vi "Lens voltage control (temp).vi"() -> ()   [LabVIEW 2018]
uses:
  <vilib>/Analysis/NI_AALBase.lvlib
  <vilib>/Analysis/baseanly.llb/Mean (DBL).vi
  <vilib>/Utility/file.llb/Write Delimited Spreadsheet (DBL).vi
panel:
  out "Scan Rate (Hz)":dbl=60.0
  out "Error Message":string
  out "Actual ScanRate":dbl format="%.3f"
  out "size(s)":i32[](array[numeric])
  out "Voltage divider 2 (V)":dbl
  out "Voltage divider 1 (V)":dbl
  in  "Active":bool
  out "Initial time":dbl
  in  "Save data path":path=path "C:/Documents and Settings/EDM/Desktop/all_cond_argon_20kV_1x10-4.txt"
  in  "Save data?":bool=TRUE caption="Enable"
  out "Supply 2 Current":waveform(dbl)(graph)
  out "Supply 1 Current":waveform(dbl)(graph)
  out "Supply 2 Voltage":waveform(dbl)(graph)
  out "Waveform Chart":dbl(graph)
  out "Loop iteration time":dbl
  in  "PS2 Set Voltage (kV)":dbl min=0.0 max=30.01 step=0.1 format="%.3f"
  in  "Both power supplies at\nsame voltage? (If true, \nPS1 voltage controls both supplies)":bool
  in  "Ramp time (s)":dbl
  out "relative seconds":dbl format="%_19f"
  out "time string":string
  out "date string":string
  in  "Polarity switch 2 (ON = pos)":bool
  in  "Polarity switch 1 (ON = pos)":bool
  in  "POWER":bool
  in  "Stop":bool
  out "PS2 Voltage (kV)":dbl
  out "PS1 Voltage (kV)":dbl
  in  "PS1 Set Voltage (kV)":dbl min=0.0 max=30.01 step=0.1 format="%.3f"
  out "Ramp Step Size (kV)":dbl=0.025
  in  "Ramp Threshold (kV)":dbl=0.025
  in  "Ramp Voltage?":bool
  out "Supply 1 Voltage":waveform(dbl)(graph)
  out "DeviceScanBacklog":i32
  out "LJMScanBacklog":i32=10
  out "Run Time":string="0  00:02:11" caption="Elapsed Time Text"
  out "Number of\nChannels":i32
  out "ScansPerRead":i32
  in  "Channels to Scan":string[](array[string])=["AIN0", "AIN1", "AIN2", "AIN3", "AIN4", "AIN5", "AIN6", "AIN7", "AIN8", "AIN9", "AIN10", "AIN11", "AIN12", "AIN13"]
  in  "Device type":string(combo)="Ethernet"
  in  "Connection Type":string(combo)="Ethernet"
  out "Connection Error on Start?":bool
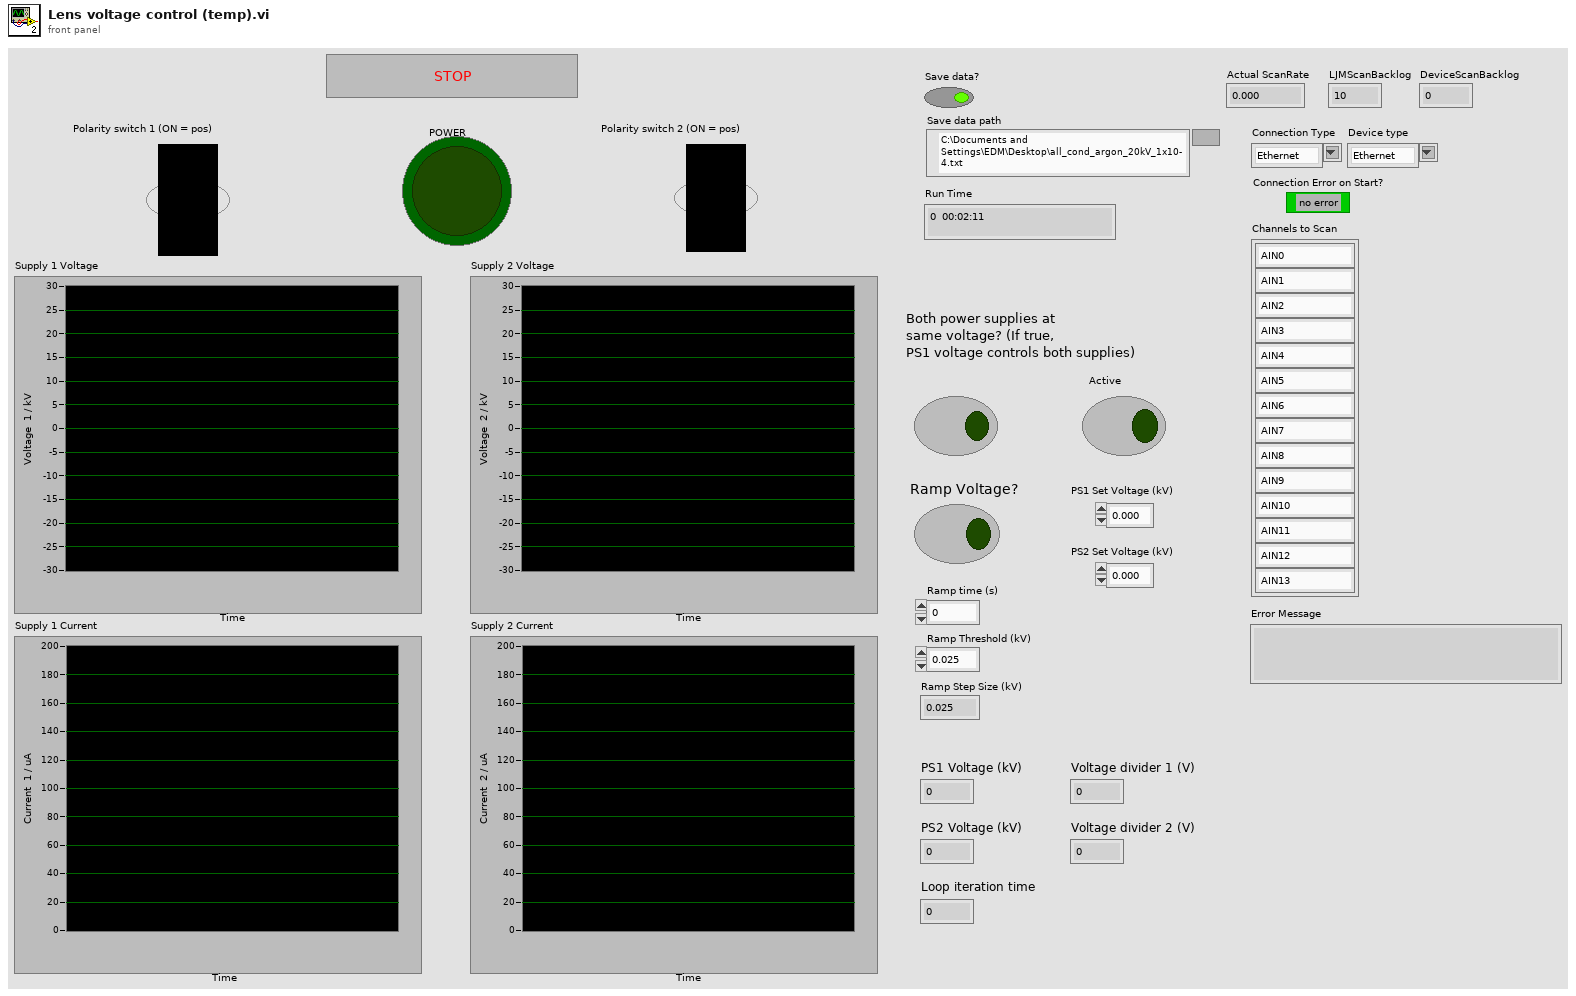
[diagram p1: front panel]
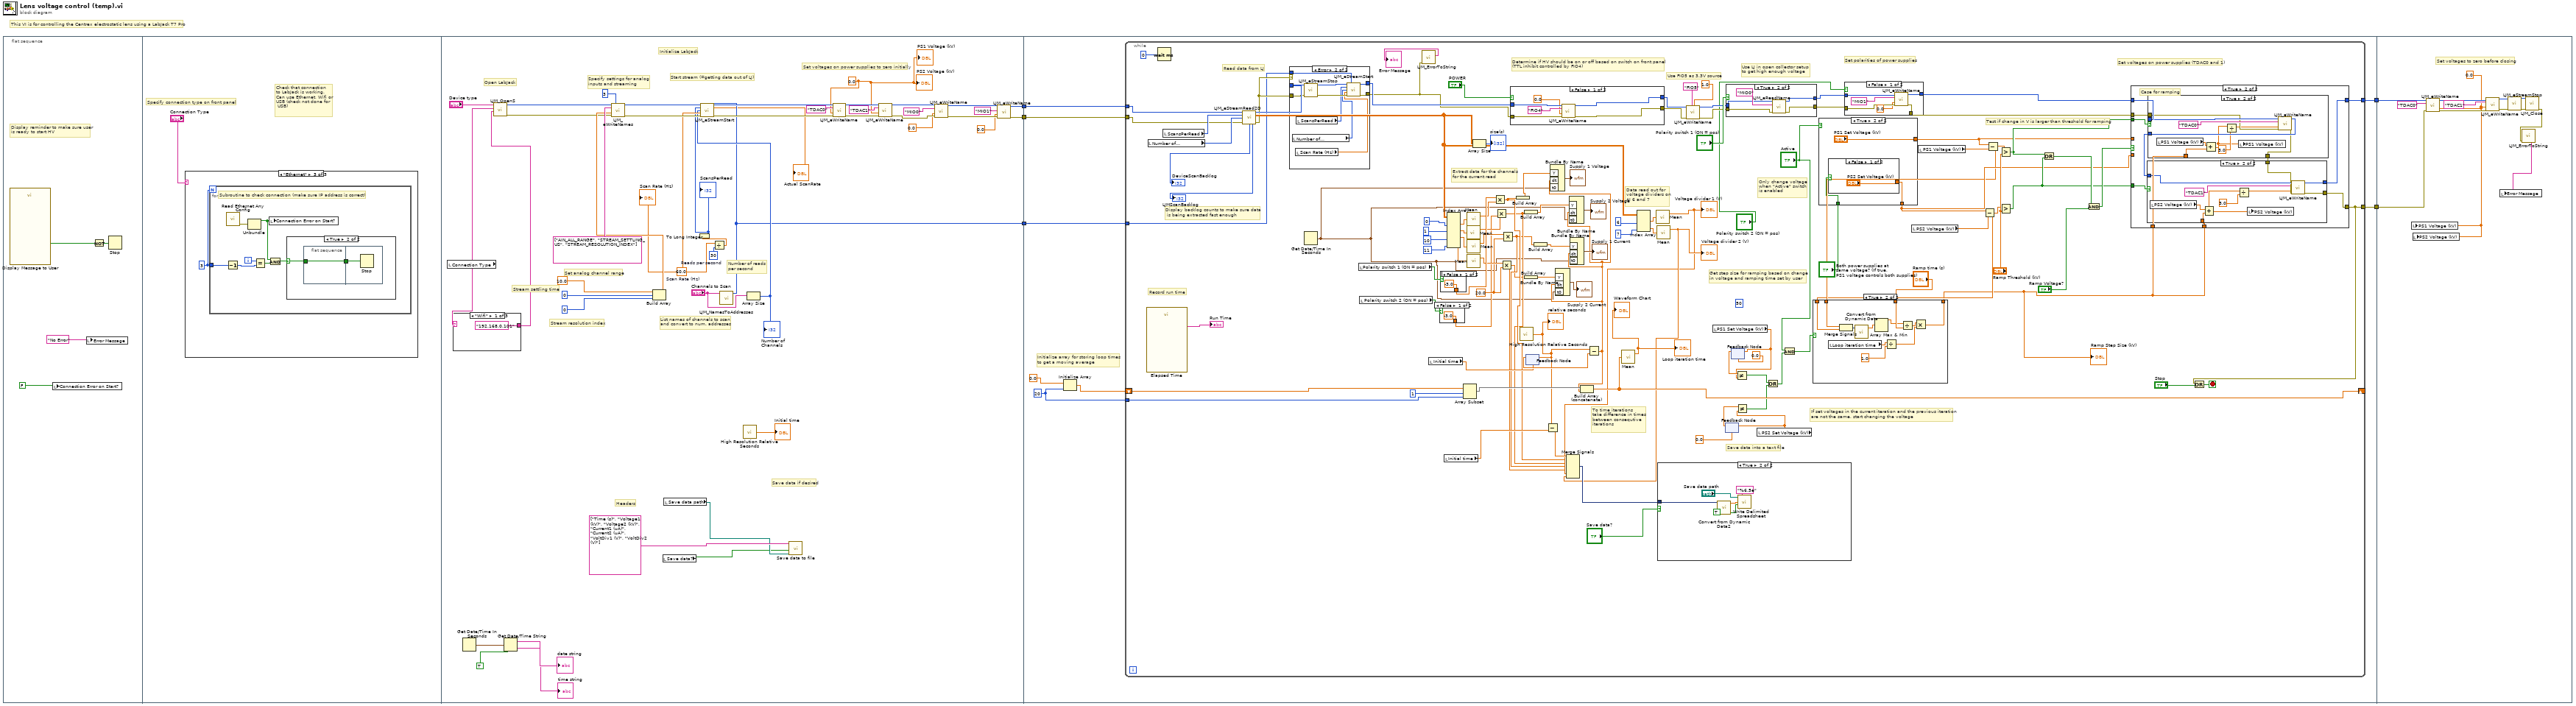
[diagram p0: block diagram]
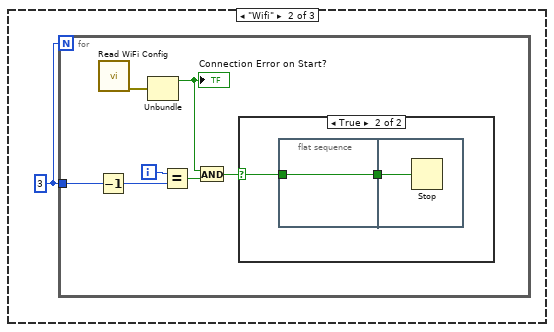
[diagram p3: hidden frame]
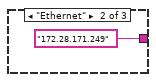
[diagram p6: hidden frame]
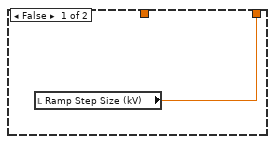
[diagram p9: hidden frame]
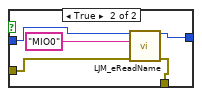
[diagram p10: hidden frame]
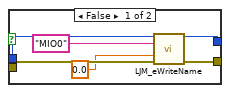
[diagram p11: hidden frame]
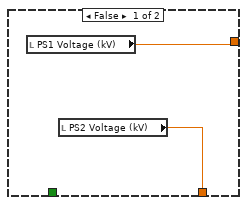
[diagram p12: hidden frame]
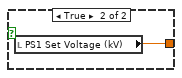
[diagram p13: hidden frame]
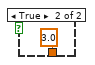
[diagram p14: hidden frame]
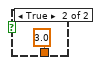
[diagram p15: hidden frame]
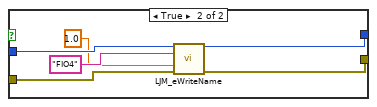
[diagram p17: hidden frame]
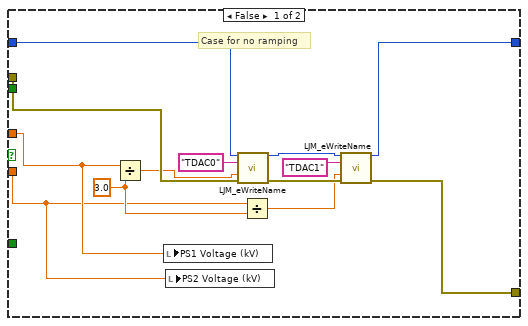
[diagram p18: hidden frame]
diagram:
  # "This VI is for controlling the Centrex electrostatic lens using a LabJack T7 Pro"
  n1 = flat-sequence {
    tunnel: [w47] -> w5
    tunnel: [w46] -> w4
    tunnel: [w40] -> w1
    tunnel: w5 -> [w90]
    tunnel: w4 -> [w89]
    tunnel: [w88] -> w3
    tunnel: [w87] -> w2
    tunnel: w1 -> [w83]
    tunnel: w3 -> [w333]
    tunnel: w2 -> [w332]
    frame #0 {
      # "Display reminder to make sure user\nis ready to start HV"
      n2 = call "Display Message to User"() -> ("GO GO GO!"=w8:bool)  [unwired: 10 in, 1 out]
      n3 = local write "Connection Error on Start?"(FALSE) -> ()
      n4 = local write "Error Message"("No Error" ("Error Message")) -> ()
      n5 = Not(x=w8) -> (.not. x?=w9:bool)
      n6 = Stop(stop? (T)=w9) -> ()
    }
    frame #1 {
      # "Specify connection type on front panel"
      # "Check that connection\nto LabJack is working.\nCan use Ethernet, Wifi or\nUSB (check not done for\n USB)"
      n7 = case shown="\"Ethernet\"" "Connection Type" {
        frame Default {
        }
        frame "Wifi" {
          w11 = 3
          n8 = for {
            N: w11 -> [_]
            tunnel: w11 -> [w13]
            i -> [w15]
            n9 = Decrement(x=w13) -> (x-1=w12:i32)
            n10 = call "Read WiFi Config.vi"() -> ("error out"=w18:errorcluster)  [unwired: 11 in]
            n11 = Unbundle(w18) -> ("status"=w17:bool)  [unwired: 2 out]
            "Connection Error on Start?" <- w17
            n12 = Equal?(x=w15, y=w12) -> (x = y?=w16:bool)
            n13 = And(x=w17, y=w16) -> (x .and. y?=w14:bool)
            n14 = case shown="True" w14 {
              selector: w14 -> [_ w20]
              frame False {
              }
              frame True {
                n15 = flat-sequence {
                  tunnel: w20 -> [w21]
                  tunnel: [w21] -> w19
                  tunnel: w19 -> [w22]
                  frame #0 {
                  }
                  frame #1 {
                    n16 = Stop(stop? (T)=w22) -> ()
                  }
                }
              }
            }
          }
        }
        frame "Ethernet" {
          w23 = 3
          n17 = for {
            N: w23 -> [_]
            tunnel: w23 -> [w27]
            i -> [w29]
            # "Subroutine to check connection (make sure IP address is correct)"
            n18 = Decrement(x=w27) -> (x-1=w26:i32)
            n19 = call "Read Ethernet Any Config.vi"() -> ("error out"=w25:errorcluster)  [unwired: 11 in]
            n20 = Unbundle(w25) -> ("status"=w24:bool)  [unwired: 2 out]
            n21 = Equal?(x=w29, y=w26) -> (x = y?=w30:bool)
            n22 = And(x=w24, y=w30) -> (x .and. y?=w28:bool)
            n23 = local write "Connection Error on Start?"(w24) -> ()
            n24 = case shown="True" w28 {
              selector: w28 -> [_ w32]
              frame False {
              }
              frame True {
                n25 = flat-sequence {
                  tunnel: w32 -> [w33]
                  tunnel: [w33] -> w31
                  tunnel: w31 -> [w34]
                  frame #0 {
                  }
                  frame #1 {
                    n26 = Stop(stop? (T)=w34) -> ()
                  }
                }
              }
            }
          }
        }
      }
    }
    frame #2 {
      w68 = 60.0  # Scan Rate (Hz)
      w45 = 0.0
      w67 = 30  # Reads per second
      # "Number of reads\nper second"
      # "Save data if desired"
      # "Headers"
      # "Stream resolution index"
      # "Stream settling time"
      # "Set analog channel range"
      # "Set voltages on power supplies to zero initially"
      # "List names of channels to scan\nand convert to num. addresses"
      # "Start stream (=getting data out of LJ)"
      # "Specify settings for analog \ninputs and streaming"
      # "Open LabJack"
      # "Initialize LabJack"
      n27 = local read "Connection Type"() -> (w79:string)
      n28 = case shown="\"Wifi\"" w79 {
        tunnel: ["192.168.0.101" "172.28.171.249" _] -> w80
        frame "Wifi" {
        }
        frame "Ethernet" {
        }
        frame Default {
        }
      }
      n29 = Get Date/Time In Seconds() -> (seconds since 1Jan1904=w38:timestamp)
      n30 = call "LJM_OpenS.vi"("Identifier"=w80, "ConnectionType"=w79, "DeviceType"="Device type") -> ("error out"=w71:errorcluster, "Handle"=w72:i32)  [unwired: 7 in]
      n31 = Get Date/Time String(seconds (now)=w38, want seconds? (F)=TRUE) -> (date string=→"date string":string, time string=→"time string":string)  [unwired: 1 in]
      n32 = Build Array(10.0 ("Analog In Range (V)"), 0 ("Stream Settling Time (us)"), 0 ("Stream Resolution Index")) -> (w73:dbl[])
      n33 = call "LJM_eWriteNames.vi"("Handle In"=w72, "NumFrames"=3, "aNames"=string[] ["AIN_ALL_RANGE", "STREAM_SETTLING_US", "STREAM_RESOLUTION_INDEX"], "aValuesIn"=w73, "error in"=w71) -> ("Handle Out"=w64:i32, "error out"=w69:errorcluster)  [unwired: 8 in, 1 out]
      n34 = local read "Save data?"() -> (w35:bool)
      n35 = local read "Save data path"() -> (w36:path)
      n36 = Divide(x=w68, y=w67) -> (x/y=w66:dbl)
      n37 = To Long Integer(number=w66) -> (32bit integer=w65:i32)
      "ScansPerRead" <- w65
      n38 = call "LJM_NamesToAddresses.vi"("aNames"="Channels to Scan") -> ("aAddresses"=w40:i32[])  [unwired: 8 in, 2 out]
      n39 = call <vilib>:"High Resolution Relative Seconds.vi"() -> ("relative seconds"=→"Initial time":dbl)
      n40 = Array Size(array="Channels to Scan") -> (size(s)=w62:i32)
      "Number of\nChannels" <- w62
      n41 = call "LJM_eStreamStart.vi"("Handle In"=w64, "aScanList"=w40, "ScansPerRead"=w65, "NumAddresses"=w62, "ScanRate"=w68, "error in"=w69) -> ("Handle Out"=w61:i32, "Actual ScanRate"=→"Actual ScanRate":dbl, "error out"=w60:errorcluster)  [unwired: 7 in]
      n42 = call "Save data to file.vi"("File path"=w36, "Save data?"=w35, "Data"=string[] ["Time (s)", "Voltage1 (kV)", "Voltage2 (kV)", "Current1 (uA)", "Current2 (uA)", "VoltDiv1 (V)", "VoltDiv2 (V)"]) -> ()  [unwired: 9 in]
      n43 = call "LJM_eWriteName.vi"("Handle In"=w61, "Name"="TDAC0", "Value"=w45, "error in"=w60) -> ("Handle Out"=w57:i32, "error out"=w58:errorcluster)  [unwired: 10 in]
      n44 = call "LJM_eWriteName.vi"("Handle In"=w57, "Name"="TDAC1", "Value"=w45, "error in"=w58) -> ("Handle Out"=w54:i32, "error out"=w55:errorcluster)  [unwired: 10 in]
      n45 = call "LJM_eWriteName.vi"("Handle In"=w54, "Name"="MIO0", "Value"=0.0, "error in"=w55) -> ("Handle Out"=w53:i32, "error out"=w50:errorcluster)  [unwired: 10 in]
      n46 = call "LJM_eWriteName.vi"("Handle In"=w53, "Name"="MIO1", "Value"=0.0, "error in"=w50) -> ("Handle Out"=w47:i32, "error out"=w46:errorcluster)  [unwired: 10 in]
      "PS1 Voltage (kV)" <- w45
      "PS2 Voltage (kV)" <- w45
      "Scan Rate (Hz)" <- w68
    }
    frame #3 {
      w84 = 20
      # "Initialize array for storing loop times\nto get a moving average"
      n47 = Initialize Array(0.0, w84) -> (w85:dbl[])
      n48 = while {
        tunnel: w90 -> [w114]
        tunnel: w89 -> [w111]
        tunnel: [w185] -> w88
        tunnel: [w106] -> w87
        shift-right: [w182] -> _
        shift-left: w85 -> [w180]
        tunnel: w84 -> [w177]
        tunnel: w83 -> [w108]
        stop <- w105 stop-if-true
        w169 = 20.0
        (unwired) 50
        # "If set voltages in the current iteration and the previous iteration\nare not the same, start changing the voltage"
        # "Use LJ in open collector setup\nto get high enough voltage"
        # "Only change voltage\nwhen \"Active\" switch\nis enabled"
        # "Set polarities of power supplies"
        # "Use FIO5 as 3.3V source"
        # "To time iterations\ntake difference in times\nbetween consequtive\niterations"
        # "Save data into a text file"
        # "Data read out for \nvoltage dividers on\nAI 6 and 7"
        # "Get step size for ramping based on change\nin voltage and ramping time set by user"
        # "Determine if HV should be on or off based on switch on front panel\n(TTL inhibit controlled by FIO4)"
        # "Test if change in V is larger than threshold for ramping"
        # "Set voltages on power supplies (TDAC0 and 1)"
        # "Extract data for the channels\nfor the current read"
        # "Display backlog counts to make sure data\n is being extracted fast enough"
        # "Record run time"
        # "Read data from LJ"
        n49 = call "Elapsed Time"() -> ("Elapsed Time Text"=→"Run Time":string)  [unwired: 12 in, 7 out]
        n50 = local read "Number of\nChannels"() -> (w197:i32)
        n51 = Wait (ms)(milliseconds to wait=0) -> ()  [unwired: 1 out]
        n52 = local read "ScansPerRead"() -> (w198:i32)
        n53 = call "LJM_eStreamRead2D.vi"("Handle In"=w114, "ScansPerRead"=w198, "NumAddresses"=w197, "error in"=w111) -> ("Handle Out"=w113:i32, "aData Out"=w153:dbl[][], "DeviceScanBacklog"=→"DeviceScanBacklog":i32, "LJMScanBacklog"=→"LJMScanBacklog":i32, "error out"=w110:errorcluster)  [unwired: 7 in]
        n54 = case shown="Error" w110 {
          tunnel: w110 -> [w200 w208]
          tunnel: [w200 w207] -> w109
          tunnel: w113 -> [w201 w209]
          tunnel: [w201 w206] -> w112
          tunnel: w108 -> [_ w202]
          frame No Error {
          }
          frame Error {
            n55 = local read "Number of\nChannels"() -> (w204:i32)
            n56 = local read "Scan Rate (Hz)"() -> (w203:dbl)
            n57 = local read "ScansPerRead"() -> (w205:i32)
            n58 = call "LJM_eStreamStop.vi"("Handle In"=w209, "error in"=w208) -> ("Handle Out"=w210:i32, "error out"=w211:errorcluster)  [unwired: 12 in]
            n59 = call "LJM_eStreamStart.vi"("Handle In"=w210, "aScanList"=w202, "ScansPerRead"=w205, "NumAddresses"=w204, "ScanRate"=w203, "error in"=w211) -> ("Handle Out"=w206:i32, "error out"=w207:errorcluster)  [unwired: 7 in, 1 out]
          }
        }
        n60 = Get Date/Time In Seconds() -> (seconds since 1Jan1904=w91:timestamp)
        n61 = local read "Polarity switch 1 (ON = pos)"() -> (w161:bool)
        n62 = local read "Polarity switch 2 (ON = pos)"() -> (w160:bool)
        n63 = call "LJM_ErrorToString.vi"("error in"=w109) -> ("String"=→"Error Message":string)  [unwired: 10 in]
        n64 = local read "Initial time"() -> (w145:dbl)
        n65 = case shown="False" w160 {
          tunnel: [-3.0 3.0] -> w159
          frame False {
          }
          frame True {
          }
        }
        n66 = case shown="False" w161 {
          tunnel: [-3.0 3.0] -> w172
          frame False {
          }
          frame True {
          }
        }
        n67 = local read "Initial time"() -> (w162:dbl)
        n68 = Index Array(array=w153, index (col) #1=0, index (col) #2=1, index (col) #3=10, index (col) #4=11) -> (element #1=w184:dbl[], element #2=w176:dbl[], element #3=w175:dbl[], element #4=w174:dbl[])  [unwired: 4 in]
        n69 = Array Subset(array=w180, index=1, length=w177) -> (w179:dbl[])
        n70 = call-poly <vilib>:"Mean.vi"("X"=w176) -> ("mean"=w167:dbl)  [unwired: 1 out]
        n71 = call-poly <vilib>:"Mean.vi"("X"=w184) -> ("mean"=w168:dbl)  [unwired: 1 out]
        n72 = call-poly <vilib>:"Mean.vi"("X"=w175) -> ("mean"=w171:dbl)  [unwired: 1 out]
        n73 = call-poly <vilib>:"Mean.vi"("X"=w174) -> ("mean"=w170:dbl)  [unwired: 1 out]
        n74 = Array Size(array=w153) -> (size(s)=→"size(s)":i32[])
        n75 = Multiply(x=w172, y=w168) -> (x*y=w103:dbl)
        n76 = Multiply(x=w167, y=w159) -> (x*y=w101:dbl)
        n77 = Multiply(x=w170, y=w169) -> (x*y=w94:dbl)
        n78 = Multiply(x=w171, y=w169) -> (x*y=w99:dbl)
        n79 = case shown="False" "POWER" {
          tunnel: w112 -> [w266 w272]
          tunnel: [w262 w269] -> w142
          tunnel: w109 -> [w265 w271]
          tunnel: [w263 w268] -> w143
          frame False {
            n80 = call "LJM_eWriteName.vi"("Handle In"=w266, "Name"="FIO4", "Value"=0.0, "error in"=w265) -> ("Handle Out"=w263:i32, "error out"=w262:errorcluster)  [unwired: 10 in]
          }
          frame True {
            n81 = call "LJM_eWriteName.vi"("Handle In"=w272, "Name"="FIO4", "Value"=1.0, "error in"=w271) -> ("Handle Out"=w268:i32, "error out"=w269:errorcluster)  [unwired: 10 in]
          }
        }
        n82 = Build Array(w103) -> (w102:dbl[])
        n83 = call <vilib>:"High Resolution Relative Seconds.vi"() -> ("relative seconds"=w166:dbl)
        "relative seconds" <- w166
        n84 = Build Array(w101) -> (w100:dbl[])
        n85 = Build Array(w94) -> (w93:dbl[])
        n86 = feedback-in #1(w166) -> ()
        n87 = feedback #1(w145) -> (w183:dbl)
        n88 = Build Array(w99) -> (w98:dbl[])
        n89 = Subtract(x=w166, y=w162) -> (x-y=w163:dbl)
        n90 = Subtract(x=w166, y=w183) -> (x-y=w92:dbl)
        n91 = Bundle By Name("Y"=w102, "dt"=w92, "t0"=w91) -> (→"Supply 1 Voltage":waveform(dbl))  [unwired: 1 in]
        n92 = Bundle By Name("Y"=w93, "dt"=w92, "t0"=w91) -> (→"Supply 2 Current":waveform(dbl))  [unwired: 1 in]
        n93 = Bundle By Name("Y"=w100, "dt"=w92, "t0"=w91) -> (→"Supply 2 Voltage":waveform(dbl))  [unwired: 1 in]
        n94 = Bundle By Name("Y"=w98, "dt"=w92, "t0"=w91) -> (→"Supply 1 Current":waveform(dbl))  [unwired: 1 in]
        n95 = Build Array (concatenate)(w179, w92) -> (w182:dbl[])
        n96 = call-poly <vilib>:"Mean.vi"("X"=w182) -> ("mean"=→"Loop iteration time" →"Waveform Chart":dbl)  [unwired: 1 out]
        n97 = Index Array(array=w153, index (col) #1=6, index (col) #2=7) -> (element #1=w155:dbl[], element #2=w154:dbl[])  [unwired: 2 in]
        n98 = call-poly <vilib>:"Mean.vi"("X"=w155) -> ("mean"=w139:dbl)  [unwired: 1 out]
        "Voltage divider 1 (V)" <- w139
        n99 = call-poly <vilib>:"Mean.vi"("X"=w154) -> ("mean"=w140:dbl)  [unwired: 1 out]
        "Voltage divider 2 (V)" <- w140
        n100 = Merge Signals(w163, w103, w101, w99, w94, w139, w140) -> (w164:dynamicdata)
        n101 = case shown="True" "Save data?" {
          tunnel: w164 -> [_ w260]
          frame False {
          }
          frame True {
            n102 = call "Convert from Dynamic Data2"("Dynamic Data Type"=w260) -> ("Array"=w259:dbl[])  [unwired: 3 in]
            n103 = call-poly <vilib>:"Write Delimited Spreadsheet.vi"("file path (dialog if empty)"="Save data path", "format (%.3f)"="%6.5e", "1D data"=w259, "append to file? (new file:F)"=TRUE) -> ()  [unwired: 10 in, 2 out]
          }
        }
        n104 = call "LJM_eWriteName.vi"("Handle In"=w143, "Name"="FIO5", "Value"=1.0, "error in"=w142) -> ("Handle Out"=w137:i32, "error out"=w136:errorcluster)  [unwired: 10 in]
        n105 = local read "PS1 Set Voltage (kV)"() -> (w118:dbl)
        n106 = feedback #2(0.0) -> (w117:dbl)
        n107 = case shown="True" "Polarity switch 1 (ON = pos)" {
          tunnel: w137 -> [w240 w244]
          tunnel: w136 -> [w239 w243]
          tunnel: [w238 w241] -> w134
          tunnel: [w237 w242] -> w133
          frame False {
            n108 = call "LJM_eWriteName.vi"("Handle In"=w240, "Name"="MIO0", "Value"=0.0, "error in"=w239) -> ("Handle Out"=w238:i32, "error out"=w237:errorcluster)  [unwired: 10 in]
          }
          frame True {
            n109 = call "LJM_eReadName.vi"("Handle In"=w244, "Name"="MIO0", "error in"=w243) -> ("Handle Out"=w241:i32, "error out"=w242:errorcluster)  [unwired: 10 in, 1 out]
          }
        }
        n110 = feedback-in #3(w118) -> ()
        n111 = feedback #3(0.0) -> (w119:dbl)
        n112 = Not Equal?(x=w119, y=w118) -> (x != y?=w128:bool)
        n113 = local read "PS2 Set Voltage (kV)"() -> (w116:dbl)
        n114 = feedback-in #2(w116) -> ()
        n115 = Not Equal?(x=w117, y=w116) -> (x != y?=w127:bool)
        n116 = Or(x=w128, y=w127) -> (x .or. y?=w126:bool)
        n117 = And(x="Active", y=w126) -> (x .and. y?=w130:bool)
        n118 = case shown="True" "Active" {
          tunnel: [w247 "PS1 Set Voltage (kV)"] -> w158
          tunnel: "Both power supplies at\nsame voltage? (If true, \nPS1 voltage controls both supplies)" -> [_ w249]
          tunnel: [w246 w248] -> w156
          frame False {
            n119 = local read "PS1 Voltage (kV)"() -> (w247:dbl)
            n120 = local read "PS2 Voltage (kV)"() -> (w246:dbl)
          }
          frame True {
            n121 = case shown="False" w249 {
              tunnel: ["PS2 Set Voltage (kV)" w252] -> w248
              frame False {
              }
              frame True {
                n122 = local read "PS1 Set Voltage (kV)"() -> (w252:dbl)
              }
            }
          }
        }
        n123 = case shown="False" "Polarity switch 2 (ON = pos)" {
          tunnel: w134 -> [w229 w233]
          tunnel: w133 -> [w227 w230]
          tunnel: [w226 w232] -> w132
          tunnel: [w225 w231] -> w131
          frame False {
            n124 = call "LJM_eWriteName.vi"("Handle In"=w229, "Name"="MIO1", "Value"=0.0, "error in"=w227) -> ("Handle Out"=w226:i32, "error out"=w225:errorcluster)  [unwired: 10 in]
          }
          frame True {
            n125 = call "LJM_eReadName.vi"("Handle In"=w233, "Name"="MIO0", "error in"=w230) -> ("Handle Out"=w232:i32, "error out"=w231:errorcluster)  [unwired: 10 in, 1 out]
          }
        }
        n126 = local read "PS2 Voltage (kV)"() -> (w190:dbl)
        n127 = local read "PS1 Voltage (kV)"() -> (w191:dbl)
        n128 = Subtract(x=w156, y=w190) -> (x-y=w124:dbl)
        n129 = Subtract(x=w158, y=w191) -> (x-y=w125:dbl)
        n130 = case shown="True" w130 {
          tunnel: w125 -> [_ w223]
          tunnel: w124 -> [_ w222]
          tunnel: "Ramp time (s)" -> [_ w221]
          tunnel: [w212 w219] -> w122
          frame False {
            n131 = local read "Ramp Step Size (kV)"() -> (w212:dbl)
          }
          frame True {
            n132 = local read "Loop iteration time"() -> (w216:dbl)
            n133 = Merge Signals(w223, w222) -> (w218:dynamicdata)
            n134 = call "Convert from Dynamic Data"("Dynamic Data Type"=w218) -> ("Array"=w217:dbl[])  [unwired: 3 in]
            n135 = Array Max & Min(array=w217) -> (max value=w215:dbl)  [unwired: 3 out]
            n136 = Divide(x=w216, y=1.0) -> (x/y=w213:dbl)
            n137 = Divide(x=w215, y=w221) -> (x/y=w214:dbl)
            n138 = Multiply(x=w214, y=w213) -> (x*y=w219:dbl)
          }
        }
        "Ramp Step Size (kV)" <- w122
        n139 = Greater?(x=w125, y="Ramp Threshold (kV)") -> (0:w188:bool)
        n140 = Greater?(x=w124, y="Ramp Threshold (kV)") -> (0:w187:bool)
        n141 = Or(x=w188, y=w187) -> (x .or. y?=w192:bool)
        n142 = And(x=w192, y="Ramp Voltage?") -> (x .and. y?=w193:bool)
        n143 = case shown="True" w193 {
          tunnel: w132 -> [w285 w294]
          tunnel: w131 -> [w281 w292]
          tunnel: w156 -> [w276 _]
          tunnel: w158 -> [w277 _]
          tunnel: w188 -> [_ w296]
          tunnel: w187 -> [_ w295]
          tunnel: w122 -> [_ w290]
          tunnel: w122 -> [_ w289]
          tunnel: [w275 w288] -> w185
          tunnel: [w274 w287] -> w106
          frame False {
            w278 = 3.0
            # "Case for no ramping"
            n144 = Divide(x=w277, y=w278) -> (x/y=w279:dbl)
            n145 = local write "PS1 Voltage (kV)"(w277) -> ()
            n146 = local write "PS2 Voltage (kV)"(w276) -> ()
            n147 = call "LJM_eWriteName.vi"("Handle In"=w285, "Name"="TDAC0", "Value"=w279, "error in"=w281) -> ("Handle Out"=w283:i32, "error out"=w282:errorcluster)  [unwired: 10 in]
            n148 = Divide(x=w276, y=w278) -> (x/y=w280:dbl)
            n149 = call "LJM_eWriteName.vi"("Handle In"=w283, "Name"="TDAC1", "Value"=w280, "error in"=w282) -> ("Handle Out"=w275:i32, "error out"=w274:errorcluster)  [unwired: 10 in]
          }
          frame True {
            # "Case for ramping"
            n150 = case shown="True" w296 {
              tunnel: w294 -> [w310 w320]
              tunnel: [w310 w319] -> w293
              tunnel: w292 -> [w309 w317]
              tunnel: [w309 w316] -> w291
              tunnel: w290 -> [_ w315]
              frame False {
              }
              frame True {
                n151 = local read "PS1 Voltage (kV)"() -> (w314:dbl)
                n152 = Add(x=w314, y=w315) -> (x+y=w311:dbl)
                n153 = Divide(x=w311, y=3.0) -> (x/y=w313:dbl)
                n154 = local write "PS1 Voltage (kV)"(w311) -> ()
                n155 = call "LJM_eWriteName.vi"("Handle In"=w320, "Name"="TDAC0", "Value"=w313, "error in"=w317) -> ("Handle Out"=w319:i32, "error out"=w316:errorcluster)  [unwired: 10 in]
              }
            }
            n156 = case shown="True" w295 {
              tunnel: w293 -> [w298 w308]
              tunnel: w291 -> [w297 w307]
              tunnel: w289 -> [_ w304]
              tunnel: [w298 w303] -> w288
              tunnel: [w297 w302] -> w287
              frame False {
              }
              frame True {
                n157 = local read "PS2 Voltage (kV)"() -> (w305:dbl)
                n158 = Add(x=w305, y=w304) -> (x+y=w299:dbl)
                n159 = Divide(x=w299, y=3.0) -> (x/y=w301:dbl)
                n160 = local write "PS2 Voltage (kV)"(w299) -> ()
                n161 = call "LJM_eWriteName.vi"("Handle In"=w308, "Name"="TDAC1", "Value"=w301, "error in"=w307) -> ("Handle Out"=w303:i32, "error out"=w302:errorcluster)  [unwired: 10 in]
              }
            }
          }
        }
        n162 = Or(x=w106, y="Stop") -> (x .or. y?=w105:bool)
      }
    }
    frame #4 {
      w327 = 0.0 ("Value")
      # "Set voltages to zero before closing"
      n163 = local write "PS1 Voltage (kV)"(w327) -> ()
      n164 = local write "PS2 Voltage (kV)"(w327) -> ()
      n165 = call "LJM_eWriteName.vi"("Handle In"=w333, "Name"="TDAC0", "Value"=w327, "error in"=w332) -> ("Handle Out"=w330:i32, "error out"=w329:errorcluster)  [unwired: 10 in]
      n166 = call "LJM_eWriteName.vi"("Handle In"=w330, "Name"="TDAC1", "Value"=w327, "error in"=w329) -> ("Handle Out"=w326:i32, "error out"=w323:errorcluster)  [unwired: 10 in]
      n167 = call "LJM_eStreamStop.vi"("Handle In"=w326, "error in"=w323) -> ("Handle Out"=w325:i32, "error out"=w324:errorcluster)  [unwired: 12 in]
      n168 = call "LJM_Close.vi"("error in"=w324, "Handle"=w325) -> ("error out"=w322:errorcluster)  [unwired: 9 in]
      n169 = call "LJM_ErrorToString.vi"("error in"=w322) -> ("String"=w321:string)  [unwired: 10 in]
      n170 = local write "Error Message"(w321) -> ()
    }
  }
